vi "Autonomous Independent.vi"() -> ()   [LabVIEW 2018]
doc: "This VI is called when autonomous begins, and will automatically be terminated when autonomous ends. You can carry out timed or sensor driven robot movement independently without needing to return to the caller."
uses:
  <vilib>/Rock Robotics/WPI/Solenoid/WPI_SolenoidValue.ctl
  <vilib>/Rock Robotics/WPI/ThirdParty/Phoenix-LabVIEW/Motor Controller/Controls/CTRE_Phoenix_MotorControl_ControlMode.ctl
  <vilib>/Rock Robotics/WPI/Utilities/WPI_GetSetVariantRefNum.vi
  <vilib>/Rock Robotics/Network Tables/NT Read String.vi
  <vilib>/Rock Robotics/Network Tables/NT Write Numeric Array.vi
  <vilib>/Rock Robotics/Network Tables/NT Read Number.vi
  <vilib>/Rock Robotics/WPI/Solenoid/WPI_SolenoidSetEnum.vi
  <vilib>/Rock Robotics/Network Tables/NT Write Boolean Array.vi
  <vilib>/Rock Robotics/WPI/RobotDrive/WPI_RobotDriveArcadeDrive_Standard(NoSaturation).vi
panel:
  in  "ScoreMode":T1(ring)
  out "Current Movement, for debugging":T2 {"Y Joystick Value" scale=1.0..-1.0; "X Joystick Value" scale=-1.0..1.0}
  in  "Array of robot movements":T3(array[cluster])=[{"X Joystick Value"=0.39393939393939403, "Y Joystick Value"=0.0, "Delay (sec)"=1.0, "Movement Name"="turn"}, {"X Joystick Value"=-0.3737373737373737, "Y Joystick Value"=0.0, "Delay (sec)"=1.0, "Movement Name"="turn back"}] {"Y Joystick Value" scale=1.0..-1.0; "X Joystick Value" scale=-1.0..1.0}
  # "Be sure to right-click and choose Data Operations>>Make Current Value default if you want to save the array values with the VI"
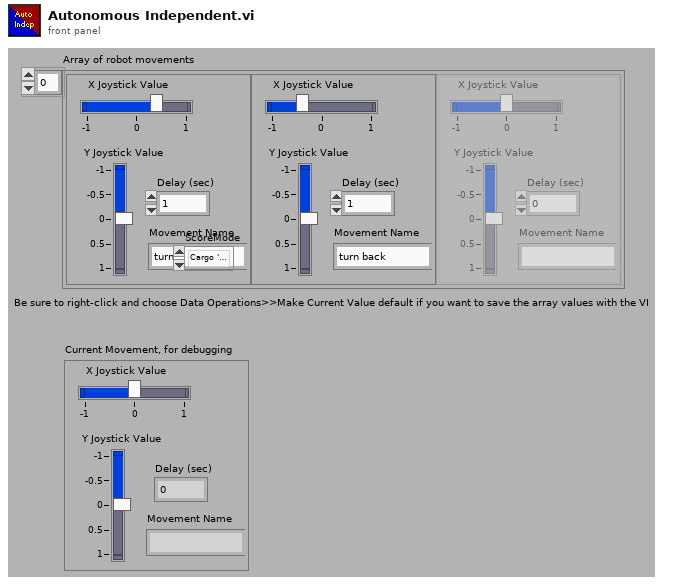
[diagram p1: front panel]
types:
  T1 = enum16{"Cargo 'default'", "Hatch", "HorseDriveHatch"}
  T2 = cluster{"X Joystick Value":dbl, "Y Joystick Value":dbl, "Delay (sec)":dbl, "Movement Name":string}
  T3 = cluster{"X Joystick Value":dbl, "Y Joystick Value":dbl, "Delay (sec)":dbl, "Movement Name":string}[]
  T4 = typedef "WPI_JoystickDevRef.ctl" = cluster{"Device":T5}
  T5 = typedef "WPI_JoystickDeviceEnum.ctl" = enum16{"USB 0", "USB 1", "USB 2", "USB 3", "USB 4", "USB 5"}
  T6 = typedef "WPI_SolenoidValue.ctl" = enum16{"Off", "On", "Forward", "Reverse"}
  T7 = typedef "CTRE_Phoenix_MotorControl_ControlMode.ctl" = u16
  T8 = typedef "WPI_MotorControlDeviceRef.ctl" = cluster{"DeviceStatus":errorcluster, "Type":T9, "PWM":cluster{"PWM Channel":T10, "DeadBand":T11}, "CAN":cluster{"Device Number":u8, "SetOutput VI Ref":variant, "GetOutput VI Ref":variant, "Enable VI Ref":variant, "Disable VI Ref":variant, "Data":variant}, "Invert":bool, "DIO PWM":cluster{"PWM \"Enable\" Channel":T10, "DIOChannel":T12, "PWM Rate":dbl}}
  T9 = typedef "WPI_MotorControlType.ctl" = enum16{"PWM", "CAN", "DIO PWM"}
  T10 = typedef "FPGA_DIOPWMChannel.ctl" = enum8{"PWM 0", "PWM 1", "PWM 2", "PWM 3", "PWM 4", "PWM 5", "PWM 6", "PWM 7", "PWM 8", "PWM 9", "PWM MXP 0", "PWM MXP 1", "PWM MXP 2", "PWM MXP 3", "PWM MXP 4", "PWM MXP 5", "PWM MXP 6", "PWM MXP 7", "PWM MXP 8", "PWM MXP 9", "Invalid"}
  T11 = typedef "WPI_PWMDeadband.ctl" = cluster{"Name":string, "maxPositivePwm":i32, "minPositivePwm":i32, "centerPwm":i32, "maxNegativePwm":i32, "minNegativePwm":i32, "angularRange":u16}
  T12 = typedef "FPGA_DIOChannel.ctl" = enum8{"DIO 0", "DIO 1", "DIO 2", "DIO 3", "DIO 4", "DIO 5", "DIO 6", "DIO 7", "DIO 8", "DIO 9", "DIO MXP 0", "DIO MXP 1", "DIO MXP 2", "DIO MXP 3", "DIO MXP 4", "DIO MXP 5", "DIO MXP 6", "DIO MXP 7", "DIO MXP 8", "DIO MXP 9", "DIO MXP 10", "DIO MXP 11", "DIO MXP 12", "DIO MXP 13", "DIO MXP 14", "DIO MXP 15", "SPI Port CS1", "SPI Port CS2", "SPI Port CS3", "SPI Port MISO", "SPI Port MOSI", "Invalid"}
  T13 = typedef "WPI_SolenoidDevRef.ctl" = cluster{"DevStatus":errorcluster, "Pneumatics Control Module":u8, "Forward Solenoid Channel":T14, "Reverse Solenoid Channel":T14}
  T14 = typedef "WPI_SolenoidChannel.ctl" = enum8{"Solenoid 0", "Solenoid 1", "Solenoid 2", "Solenoid 3", "Solenoid 4", "Solenoid 5", "Solenoid 6", "Solenoid 7", "Invalid"}
  T15 = typedef "WPI_RobotDriveDevRef.ctl" = cluster{"DevStatus":errorcluster, "Motors[]":T8[], "Square Inputs":bool, "Max Output":dbl}
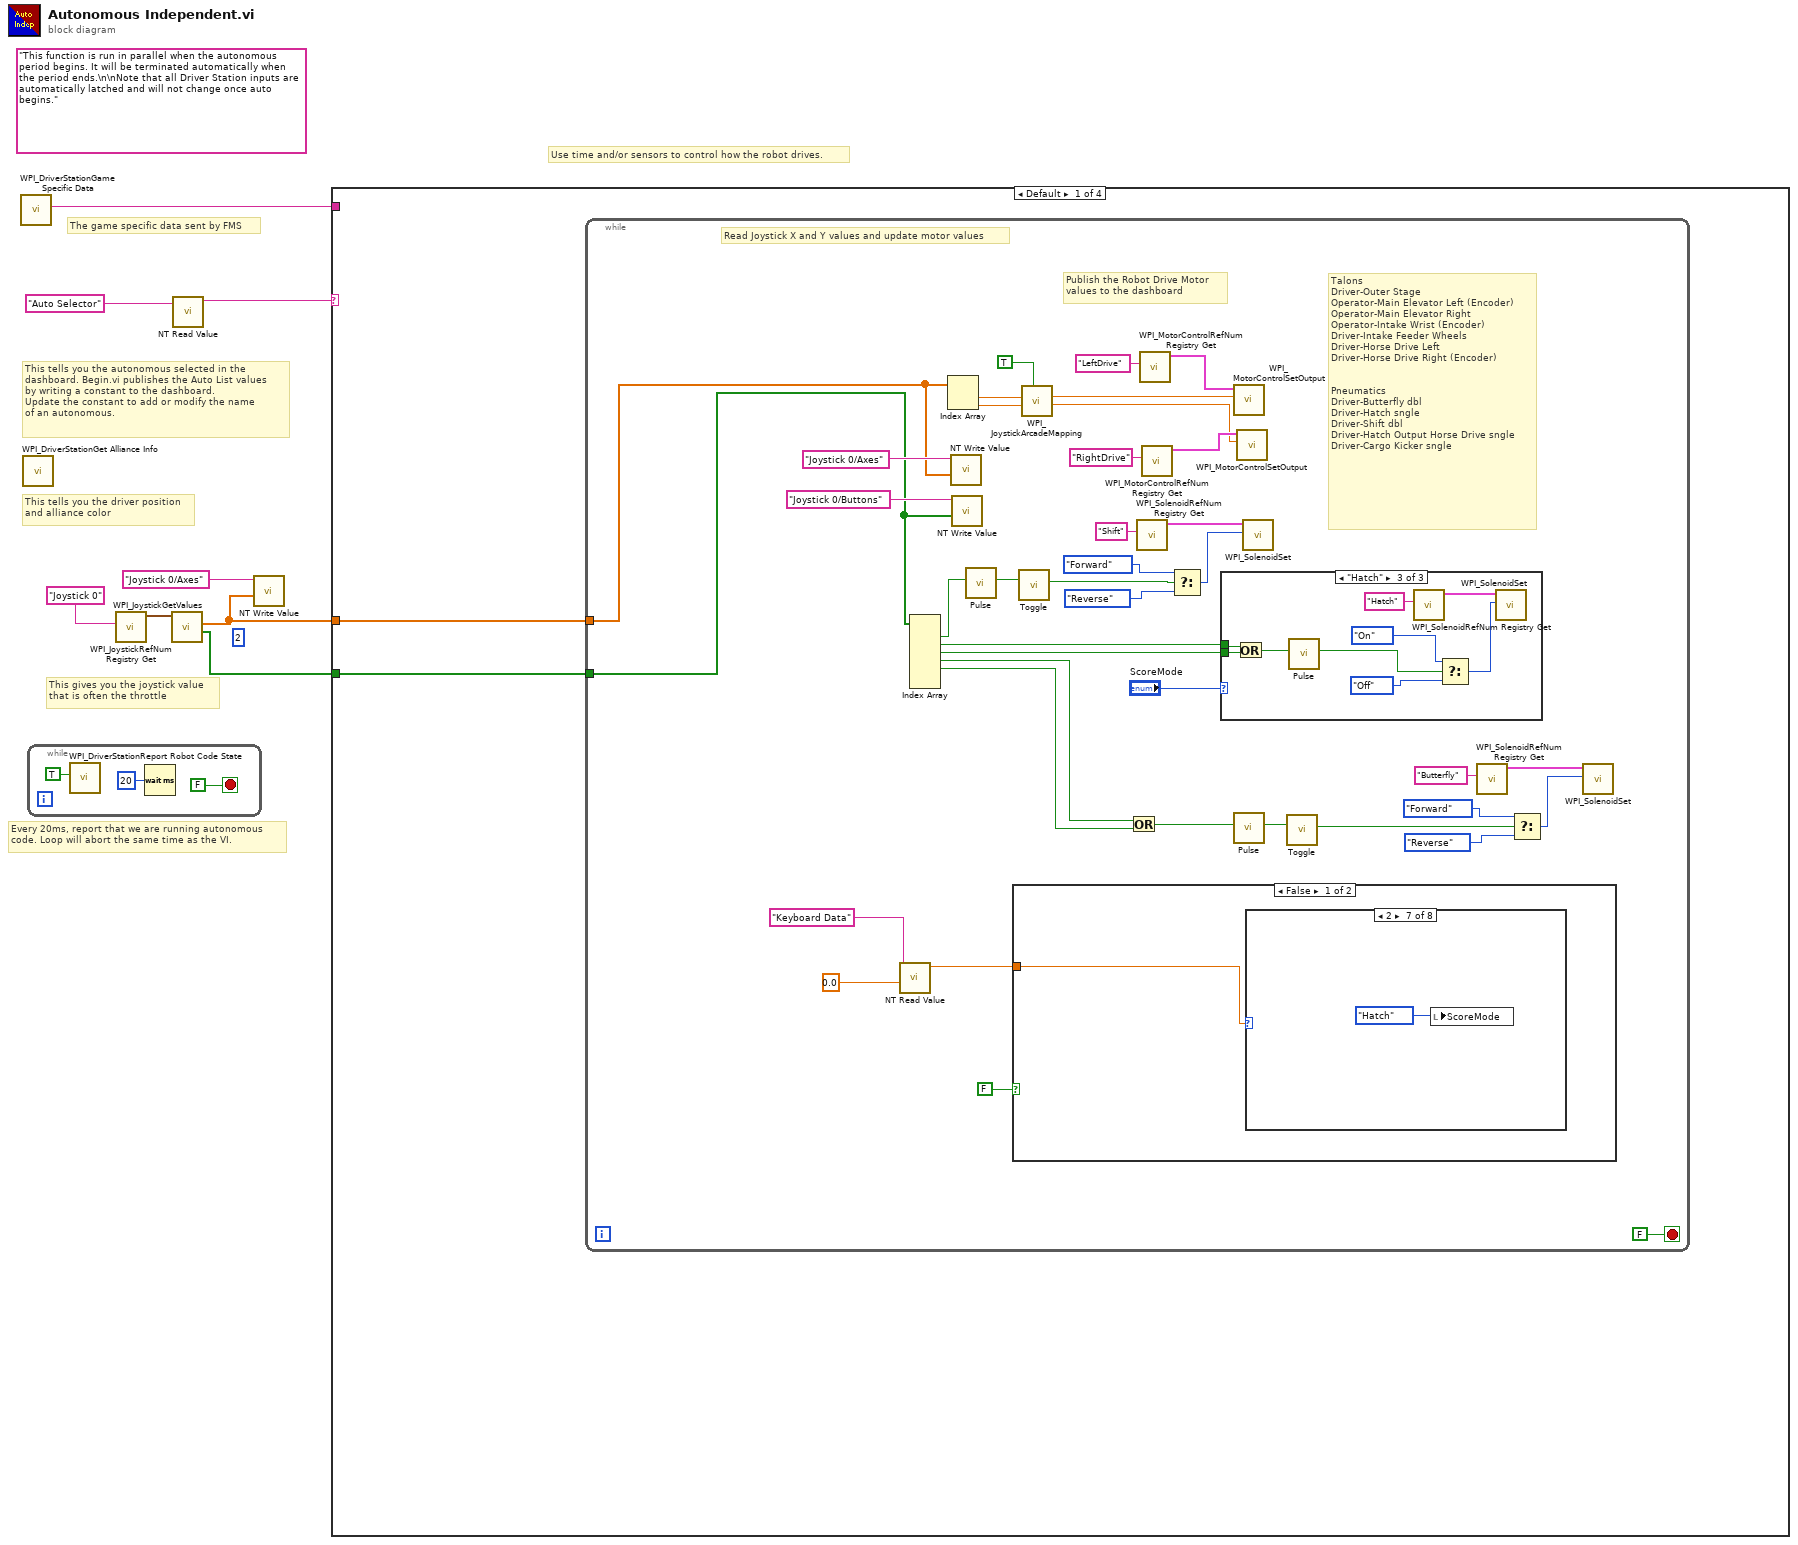
[diagram p0: block diagram]
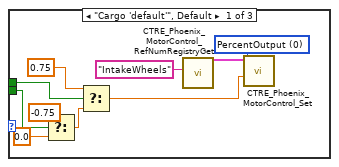
[diagram p2: hidden frame]
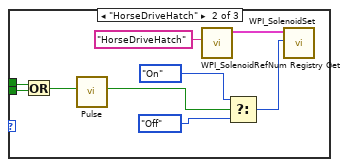
[diagram p3: hidden frame]
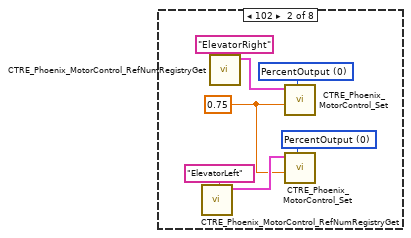
[diagram p5: hidden frame]
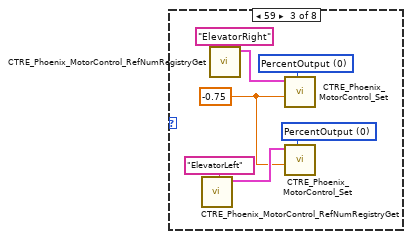
[diagram p6: hidden frame]
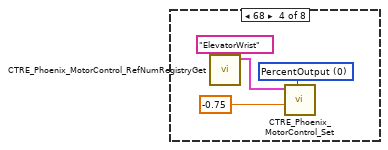
[diagram p7: hidden frame]
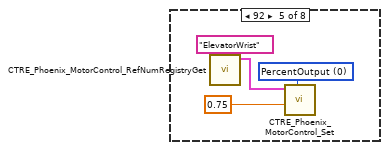
[diagram p8: hidden frame]
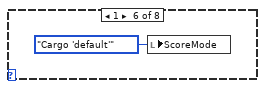
[diagram p9: hidden frame]
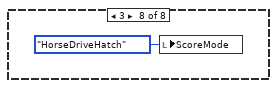
[diagram p10: hidden frame]
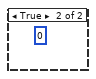
[diagram p11: hidden frame]
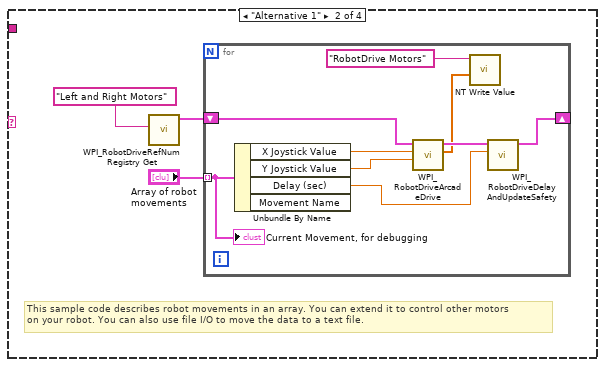
[diagram p12: hidden frame]
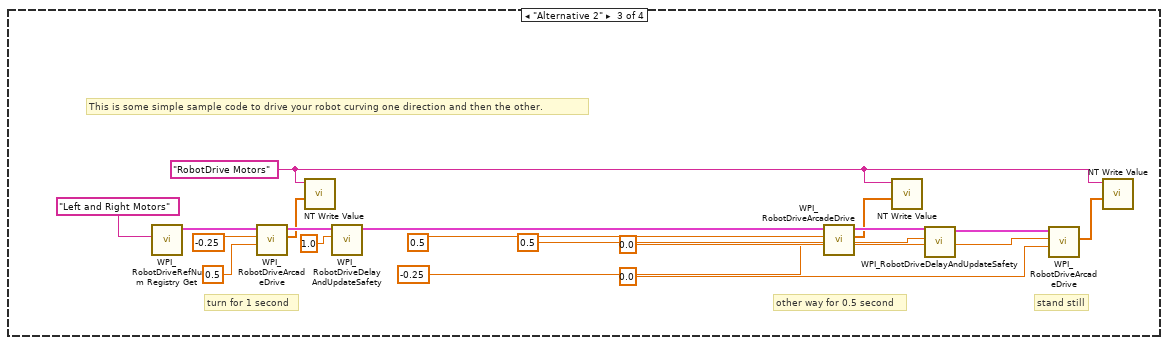
[diagram p13: hidden frame]
diagram:
  (unwired) 2 ("index")
  (unwired) "This function is run in parallel when the autonomous period begins. It will be terminated automatically when the period ends.\n\nNote that all Driver Station inputs are automatically latched and will not change once auto begins."
  # "The game specific data sent by FMS"
  # "This tells you the autonomous selected in the \ndashboard. Begin.vi publishes the Auto List values\nby writing a constant to the dashboard.\nUpdate the constant to add or modify the name\nof an autonomous."
  # "Every 20ms, report that we are running autonomous\ncode. Loop will abort the same time as the VI."
  # "This gives you the joystick value\nthat is often the throttle"
  # "Use time and/or sensors to control how the robot drives."
  # "This tells you the driver position\nand alliance color"
  n1 = call <vilib>:"WPI_DriverStationGame Specific Data.vi"() -> ("Game Specific Data"=w3:string)  [unwired: 11 in]
  n2 = call <vilib>:"WPI_DriverStationGet Alliance Info.vi"() -> ()  [unwired: 12 out]
  n3 = while {
    stop <- FALSE stop-if-true
    n4 = call <vilib>:"WPI_DriverStationReport Robot Code State.vi"("Autonomous"=TRUE) -> ()  [unwired: 10 in, 1 out]
    n5 = Wait (ms)(milliseconds to wait=u32 20) -> ()  [unwired: 1 out]
  }
  n6 = call <vilib>:"WPI_JoystickRefNum Registry Get.vi"("refnum name"="Joystick 0") -> ("JoystickDevRef"=w7:T4)  [unwired: 1 in, 9 out]
  n7 = call <vilib>:"WPI_JoystickGetValues.vi"("JoystickDevRef"=w7) -> ("Buttons"=w1:bool[], "Axes"=w2:dbl[])  [unwired: 6 in, 3 out]
  n8 = call-poly <vilib>:"NT Read Value.vi"("Name"="Auto Selector") -> ("String"=w5:string)  [unwired: 9 in, 1 out]
  n9 = call-poly <vilib>:"NT Write Value.vi"("Numeric Array"=w2, "Name"="Joystick 0/Axes") -> ()  [unwired: 9 in, 1 out]
  n10 = case shown="Default" w5 {
    tunnel: w3 -> [_ _ _ _]
    tunnel: w2 -> [w13 _ _ _]
    tunnel: w1 -> [w12 _ _ _]
    frame Default {
      n11 = while {
        tunnel: w13 -> [w16]
        tunnel: w12 -> [w15]
        stop <- FALSE stop-if-true
        # "Talons\nDriver-Outer Stage \nOperator-Main Elevator Left (Encoder)\nOperator-Main Elevator Right\nOperator-Intake Wrist (Encoder)\nDriver-Intake Feeder Wheels\nDriver-Horse Drive Left\nDriver-Horse Drive Right (Encoder)\n\n\nPneumatics\nDriver-Butterfly dbl \nDriver-Hatch sngle\nDriver-Shift dbl\nDriver-Hatch Output Horse Drive sngle\nDriver-Cargo Kicker sngle"
        # "Publish the Robot Drive Motor\nvalues to the dashboard"
        # "Read Joystick X and Y values and update motor values"
        n12 = call-poly <vilib>:"NT Read Value.vi"("Default Value"=0.0, "Name"="Keyboard Data") -> ("Numeric"=w17:dbl)  [unwired: 8 in, 1 out]
        n13 = Index Array(array=w15) -> (element #1=w37:bool, element #2=w33:bool, element #3=w32:bool, element #4=w29:bool, element #5=w28:bool)  [unwired: 7 in, 2 out]
        n14 = Index Array(array=w16) -> (element #1=w50:dbl, element #2=w49:dbl)  [unwired: 2 in]
        n15 = call-poly <vilib>:"NT Write Value.vi"("Numeric Array"=w16, "Name"="Joystick 0/Axes") -> ()  [unwired: 9 in, 1 out]
        n16 = call-poly <vilib>:"NT Write Value.vi"("Boolean Array"=w15, "Name"="Joystick 0/Buttons") -> ()  [unwired: 9 in, 1 out]
        n17 = call "Pulse.vi"("Input"=w37) -> ("Output"=w36:bool)  [unwired: 10 in]
        n18 = case shown="False" FALSE {
          tunnel: w17 -> [w81 _]
          frame False {
            n19 = case shown="2" w81 {
              frame 0, Default {
              }
              frame 102 {
                w82 = 0.75 ("Output")
                w84 = T7 0 items=["PercentOutput"=0, "Position"=1, "Velocity"=2, "Current"=3, "Follower"=5, "MotionProfile"=6, "MotionMagic"=7, "MotionProfileArc"=10, "Disabled"=15] ("Control Mode")
                w88 = T7 0 items=["PercentOutput"=0, "Position"=1, "Velocity"=2, "Current"=3, "Follower"=5, "MotionProfile"=6, "MotionMagic"=7, "MotionProfileArc"=10, "Disabled"=15] ("Control Mode")
                n20 = call <vilib>:"CTRE_Phoenix_MotorControl_RefNumRegistryGet.vi"("refnum name"="ElevatorLeft") -> ("PhoenixMotorControlDevRef"=w85:T8)  [unwired: 9 in, 1 out]
                n21 = call <vilib>:"CTRE_Phoenix_MotorControl_RefNumRegistryGet.vi"("refnum name"="ElevatorRight") -> ("PhoenixMotorControlDevRef"=w87:T8)  [unwired: 9 in, 1 out]
                n22 = call <vilib>:"CTRE_Phoenix_MotorControl_Set.vi"("Output"=w82, "Control Mode"=w88, "PhoenixMotorControlDevRef"=w87) -> ()  [unwired: 7 in, 2 out]
                n23 = call <vilib>:"CTRE_Phoenix_MotorControl_Set.vi"("Output"=w82, "Control Mode"=w84, "PhoenixMotorControlDevRef"=w85) -> ()  [unwired: 7 in, 2 out]
              }
              frame 59 {
                w89 = -0.75 ("Output")
                w91 = T7 0 items=["PercentOutput"=0, "Position"=1, "Velocity"=2, "Current"=3, "Follower"=5, "MotionProfile"=6, "MotionMagic"=7, "MotionProfileArc"=10, "Disabled"=15] ("Control Mode")
                w95 = T7 0 items=["PercentOutput"=0, "Position"=1, "Velocity"=2, "Current"=3, "Follower"=5, "MotionProfile"=6, "MotionMagic"=7, "MotionProfileArc"=10, "Disabled"=15] ("Control Mode")
                n24 = call <vilib>:"CTRE_Phoenix_MotorControl_RefNumRegistryGet.vi"("refnum name"="ElevatorLeft") -> ("PhoenixMotorControlDevRef"=w92:T8)  [unwired: 9 in, 1 out]
                n25 = call <vilib>:"CTRE_Phoenix_MotorControl_RefNumRegistryGet.vi"("refnum name"="ElevatorRight") -> ("PhoenixMotorControlDevRef"=w94:T8)  [unwired: 9 in, 1 out]
                n26 = call <vilib>:"CTRE_Phoenix_MotorControl_Set.vi"("Output"=w89, "Control Mode"=w95, "PhoenixMotorControlDevRef"=w94) -> ()  [unwired: 7 in, 2 out]
                n27 = call <vilib>:"CTRE_Phoenix_MotorControl_Set.vi"("Output"=w89, "Control Mode"=w91, "PhoenixMotorControlDevRef"=w92) -> ()  [unwired: 7 in, 2 out]
              }
              frame 68 {
                w99 = T7 0 items=["PercentOutput"=0, "Position"=1, "Velocity"=2, "Current"=3, "Follower"=5, "MotionProfile"=6, "MotionMagic"=7, "MotionProfileArc"=10, "Disabled"=15] ("Control Mode")
                n28 = call <vilib>:"CTRE_Phoenix_MotorControl_RefNumRegistryGet.vi"("refnum name"="ElevatorWrist") -> ("PhoenixMotorControlDevRef"=w98:T8)  [unwired: 9 in, 1 out]
                n29 = call <vilib>:"CTRE_Phoenix_MotorControl_Set.vi"("Output"=-0.75, "Control Mode"=w99, "PhoenixMotorControlDevRef"=w98) -> ()  [unwired: 7 in, 2 out]
              }
              frame 92 {
                w103 = T7 0 items=["PercentOutput"=0, "Position"=1, "Velocity"=2, "Current"=3, "Follower"=5, "MotionProfile"=6, "MotionMagic"=7, "MotionProfileArc"=10, "Disabled"=15] ("Control Mode")
                n30 = call <vilib>:"CTRE_Phoenix_MotorControl_RefNumRegistryGet.vi"("refnum name"="ElevatorWrist") -> ("PhoenixMotorControlDevRef"=w102:T8)  [unwired: 9 in, 1 out]
                n31 = call <vilib>:"CTRE_Phoenix_MotorControl_Set.vi"("Output"=0.75, "Control Mode"=w103, "PhoenixMotorControlDevRef"=w102) -> ()  [unwired: 7 in, 2 out]
              }
              frame 1 {
                n32 = local write "ScoreMode"(T1."Cargo 'default'" ("ScoreMode")) -> ()
              }
              frame 2 {
                n33 = local write "ScoreMode"(T1."Hatch" ("ScoreMode")) -> ()
              }
              frame 3 {
                n34 = local write "ScoreMode"(T1."HorseDriveHatch" ("ScoreMode")) -> ()
              }
            }
          }
          frame True {
            (unwired) 0
          }
        }
        n35 = call "Toggle.vi"("Input"=w36) -> ("Output"=w35:bool)  [unwired: 10 in]
        n36 = call <vilib>:"WPI_JoystickArcadeMapping.vi"("Square Inputs"=TRUE, "Y axis value"=w49, "X axis value"=w50) -> ("Right Motor Value"=w42:dbl, "Left Motor Value"=w45:dbl)  [unwired: 7 in]
        n37 = Or(x=w29, y=w28) -> (x .or. y?=w27:bool)
        n38 = call <vilib>:"WPI_SolenoidRefNum Registry Get.vi"("refnum name"="Shift") -> ("SolenoidDevRef"=w40:T13)  [unwired: 9 in, 1 out]
        n39 = call <vilib>:"WPI_MotorControlRefNum Registry Get.vi"("refnum name"="LeftDrive") -> ("MotorControlDevRef"=w47:T8)  [unwired: 9 in, 1 out]
        n40 = call <vilib>:"WPI_MotorControlRefNum Registry Get.vi"("refnum name"="RightDrive") -> ("MotorControlDevRef"=w43:T8)  [unwired: 9 in, 1 out]
        n41 = Select(t=WPI_SolenoidValue."Forward" ("Value"), s=w35, f=WPI_SolenoidValue."Reverse" ("Value")) -> (s? t:f=w34:T6)
        n42 = case shown="\"Hatch\"" "ScoreMode" {
          tunnel: w33 -> [w59 w68 w77]
          tunnel: w32 -> [w58 w69 w78]
          frame "Cargo 'default'", Default {
            w60 = T7 0 items=["PercentOutput"=0, "Position"=1, "Velocity"=2, "Current"=3, "Follower"=5, "MotionProfile"=6, "MotionMagic"=7, "MotionProfileArc"=10, "Disabled"=15] ("Control Mode")
            n43 = Select(t=-0.75, s=w58, f=0.0) -> (s? t:f=w57:dbl)
            n44 = Select(t=0.75, s=w59, f=w57) -> (s? t:f=w53:dbl)
            n45 = call <vilib>:"CTRE_Phoenix_MotorControl_RefNumRegistryGet.vi"("refnum name"="IntakeWheels") -> ("PhoenixMotorControlDevRef"=w61:T8)  [unwired: 9 in, 1 out]
            n46 = call <vilib>:"CTRE_Phoenix_MotorControl_Set.vi"("Output"=w53, "Control Mode"=w60, "PhoenixMotorControlDevRef"=w61) -> ()  [unwired: 7 in, 2 out]
          }
          frame "HorseDriveHatch" {
            n47 = Or(x=w68, y=w69) -> (x .or. y?=w67:bool)
            n48 = call "Pulse.vi"("Input"=w67) -> ("Output"=w66:bool)  [unwired: 10 in]
            n49 = call <vilib>:"WPI_SolenoidRefNum Registry Get.vi"("refnum name"="HorseDriveHatch") -> ("SolenoidDevRef"=w71:T13)  [unwired: 9 in, 1 out]
            n50 = Select(t=WPI_SolenoidValue."On" ("Value"), s=w66, f=WPI_SolenoidValue."Off" ("Value")) -> (s? t:f=w63:T6)
            n51 = call-poly <vilib>:"WPI_SolenoidSet.vi"("Value"=w63, "SolenoidDevRef"=w71) -> ()  [unwired: 8 in, 2 out]
          }
          frame "Hatch" {
            n52 = Or(x=w77, y=w78) -> (x .or. y?=w76:bool)
            n53 = call "Pulse.vi"("Input"=w76) -> ("Output"=w75:bool)  [unwired: 10 in]
            n54 = call <vilib>:"WPI_SolenoidRefNum Registry Get.vi"("refnum name"="Hatch") -> ("SolenoidDevRef"=w80:T13)  [unwired: 9 in, 1 out]
            n55 = Select(t=WPI_SolenoidValue."On" ("Value"), s=w75, f=WPI_SolenoidValue."Off" ("Value")) -> (s? t:f=w72:T6)
            n56 = call-poly <vilib>:"WPI_SolenoidSet.vi"("Value"=w72, "SolenoidDevRef"=w80) -> ()  [unwired: 8 in, 2 out]
          }
        }
        n57 = call <vilib>:"WPI_MotorControlSetOutput.vi"("Output"=w45, "MotorControlDevRef"=w47) -> ()  [unwired: 7 in, 3 out]
        n58 = call "Pulse.vi"("Input"=w27) -> ("Output"=w31:bool)  [unwired: 10 in]
        n59 = call <vilib>:"WPI_MotorControlSetOutput.vi"("Output"=w42, "MotorControlDevRef"=w43) -> ()  [unwired: 7 in, 3 out]
        n60 = call-poly <vilib>:"WPI_SolenoidSet.vi"("Value"=w34, "SolenoidDevRef"=w40) -> ()  [unwired: 8 in, 2 out]
        n61 = call "Toggle.vi"("Input"=w31) -> ("Output"=w21:bool)  [unwired: 10 in]
        n62 = call <vilib>:"WPI_SolenoidRefNum Registry Get.vi"("refnum name"="Butterfly") -> ("SolenoidDevRef"=w23:T13)  [unwired: 9 in, 1 out]
        n63 = Select(t=WPI_SolenoidValue."Forward" ("Value"), s=w21, f=WPI_SolenoidValue."Reverse" ("Value")) -> (s? t:f=w26:T6)
        n64 = call-poly <vilib>:"WPI_SolenoidSet.vi"("Value"=w26, "SolenoidDevRef"=w23) -> ()  [unwired: 8 in, 2 out]
      }
    }
    frame "Alternative 1" {
      # "This sample code describes robot movements in an array. You can extend it to control other motors\non your robot. You can also use file I/O to move the data to a text file."
      n65 = call <vilib>:"WPI_RobotDriveRefNum Registry Get.vi"("refnum name"="Left and Right Motors") -> ("RobotDriveDevRef"=w108:T15)  [unwired: 1 in, 9 out]
      n66 = for {
        shift-right: [w116] -> _
        shift-left: w108 -> [w117]
        tunnel: "Array of robot movements" -> [w112] mode=indexing
        n67 = Unbundle By Name(w112) -> ("X Joystick Value"=w115:dbl, "Y Joystick Value"=w114:dbl, "Delay (sec)"=w113:dbl)  [unwired: 1 out]
        n68 = call-poly <vilib>:"WPI_RobotDriveArcadeDrive.vi"("Y axis value"=w114, "X axis value"=w115, "RobotDriveDevRef"=w117) -> ("Motor Values"=w110:dbl[], "RobotDriveDevRef"=w118:T15)  [unwired: 1 in, 6 out]
        n69 = call-poly <vilib>:"NT Write Value.vi"("Numeric Array"=w110, "Name"="RobotDrive Motors") -> ()  [unwired: 9 in, 1 out]
        n70 = call <vilib>:"WPI_RobotDriveDelayAndUpdateSafety.vi"("Delay (s)"=w113, "RobotDriveDevRef"=w118) -> ("RobotDriveDevRef 2"=w116:T15)  [unwired: 8 in, 1 out]
        "Current Movement, for debugging" <- w112
      }
    }
    frame "Alternative 2" {
      w120 = "RobotDrive Motors" ("Name")
      # "This is some simple sample code to drive your robot curving one direction and then the other."
      # "stand still"
      # "other way for 0.5 second"
      # "turn for 1 second"
      n71 = call <vilib>:"WPI_RobotDriveRefNum Registry Get.vi"("refnum name"="Left and Right Motors") -> ("RobotDriveDevRef"=w136:T15)  [unwired: 1 in, 9 out]
      n72 = call-poly <vilib>:"WPI_RobotDriveArcadeDrive.vi"("Y axis value"=0.5 ("X axis value"), "X axis value"=-0.25, "RobotDriveDevRef"=w136) -> ("Motor Values"=w119:dbl[], "RobotDriveDevRef"=w129:T15)  [unwired: 1 in, 6 out]
      n73 = call-poly <vilib>:"NT Write Value.vi"("Numeric Array"=w119, "Name"=w120) -> ()  [unwired: 9 in, 1 out]
      n74 = call <vilib>:"WPI_RobotDriveDelayAndUpdateSafety.vi"("Delay (s)"=1.0, "RobotDriveDevRef"=w129) -> ("RobotDriveDevRef 2"=w130:T15)  [unwired: 8 in, 1 out]
      n75 = call-poly <vilib>:"WPI_RobotDriveArcadeDrive.vi"("Y axis value"=-0.25 ("X axis value"), "X axis value"=0.5, "RobotDriveDevRef"=w130) -> ("Motor Values"=w121:dbl[], "RobotDriveDevRef"=w131:T15)  [unwired: 1 in, 6 out]
      n76 = call-poly <vilib>:"NT Write Value.vi"("Numeric Array"=w121, "Name"=w120) -> ()  [unwired: 9 in, 1 out]
      n77 = call <vilib>:"WPI_RobotDriveDelayAndUpdateSafety.vi"("Delay (s)"=0.5, "RobotDriveDevRef"=w131) -> ("RobotDriveDevRef 2"=w132:T15)  [unwired: 8 in, 1 out]
      n78 = call-poly <vilib>:"WPI_RobotDriveArcadeDrive.vi"("Y axis value"=0.0 ("X axis value"), "X axis value"=0.0, "RobotDriveDevRef"=w132) -> ("Motor Values"=w122:dbl[])  [unwired: 1 in, 7 out]
      n79 = call-poly <vilib>:"NT Write Value.vi"("Numeric Array"=w122, "Name"=w120) -> ()  [unwired: 9 in, 1 out]
    }
    frame "Your Turn" {
    }
  }
